vi "坐标映射.vi"(10 "位置":enum16{"A", "B", "C", "D", "E", "F", "G", "H"}(ring)) -> (0 "差值坐标":cluster{"X":i32, "Y":i32}, 1 "O均值坐标":cluster{"X":i32, "Y":i32}, 2 "位置均值坐标":cluster{"X":i32, "Y":i32}, 3 "位置坐标":cluster{"X":i32, "Y":i32}[](array[cluster]))   [LabVIEW 2015]
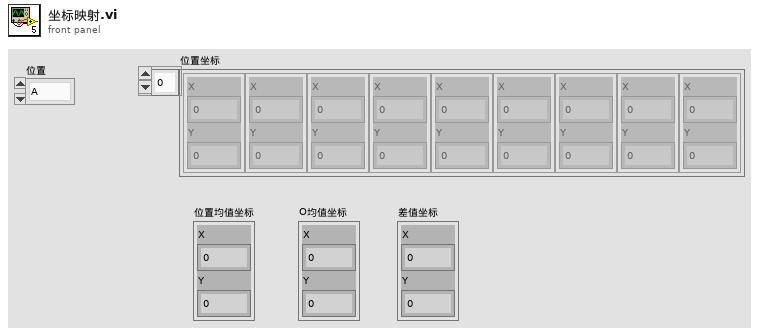
[diagram p1: front panel]
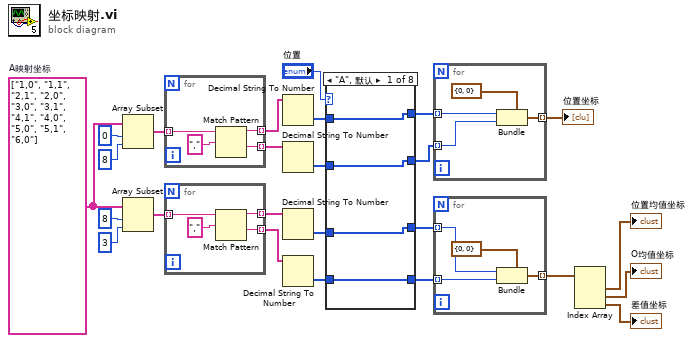
[diagram p0: block diagram]
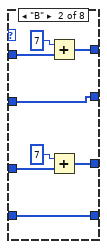
[diagram p2: hidden frame]
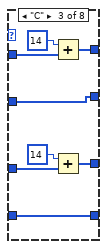
[diagram p3: hidden frame]
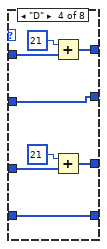
[diagram p4: hidden frame]
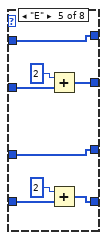
[diagram p5: hidden frame]
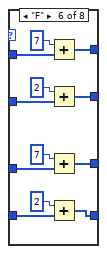
[diagram p6: hidden frame]
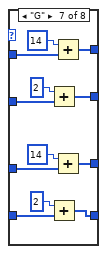
[diagram p7: hidden frame]
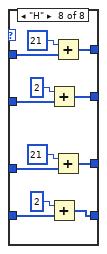
[diagram p8: hidden frame]
diagram:
  w16 = string[] ["1,0", "1,1", "2,1", "2,0", "3,0", "3,1", "4,1", "4,0", "5,0", "5,1", "6,0"]  # A映射坐标
  n1 = Array Subset(array=w16, index=0 ("索引"), length=8 ("索引")) -> (w15:string[])
  n2 = Array Subset(array=w16, index=8 ("索引"), length=3 ("索引")) -> (w14:string[])
  n3 = for {
    tunnel: w15 -> [w29] mode=indexing
    tunnel: [w27] -> w25 mode=indexing
    tunnel: [w26] -> w24 mode=indexing
    n4 = Match Pattern(string=w29, regular expression="," ("正则表达式")) -> (before substring=w27:string, after substring=w26:string)  [unwired: 1 in, 2 out]
  }
  n5 = for {
    tunnel: w14 -> [w33] mode=indexing
    tunnel: [w31] -> w13 mode=indexing
    tunnel: [w30] -> w12 mode=indexing
    n6 = Match Pattern(string=w33, regular expression="," ("正则表达式")) -> (before substring=w31:string, after substring=w30:string)  [unwired: 1 in, 2 out]
  }
  n7 = Decimal String To Number(string=w25) -> (number=w22:i32[])  [unwired: 2 in, 1 out]
  n8 = Decimal String To Number(string=w24) -> (number=w21:i32[])  [unwired: 2 in, 1 out]
  n9 = Decimal String To Number(string=w13) -> (number=w11:i32[])  [unwired: 2 in, 1 out]
  n10 = Decimal String To Number(string=w12) -> (number=w10:i32[])  [unwired: 2 in, 1 out]
  n11 = case shown="\"A\", 默认" "位置" {
    tunnel: [w37 w42 w50 w58 w69 w79 w91 w103] -> w3
    tunnel: w22 -> [w37 w44 w52 w60 w69 w81 w93 w105]
    tunnel: w21 -> [w36 w45 w53 w61 w67 w77 w89 w101]
    tunnel: [w36 w45 w53 w61 w66 w76 w88 w100] -> w2
    tunnel: w11 -> [w35 w40 w48 w56 w62 w73 w85 w97]
    tunnel: w10 -> [w34 w38 w46 w54 w64 w71 w84 w95]
    tunnel: [w35 w39 w47 w55 w62 w72 w83 w96] -> w9
    tunnel: [w34 w38 w46 w54 w63 w70 w82 w94] -> w8
    frame "A", Default {
    }
    frame "B" {
      n12 = Add(x=7, y=w44) -> (x+y=w42:i32[])
      n13 = Add(x=7, y=w40) -> (x+y=w39:i32[])
    }
    frame "C" {
      n14 = Add(x=14, y=w52) -> (x+y=w50:i32[])
      n15 = Add(x=14, y=w48) -> (x+y=w47:i32[])
    }
    frame "D" {
      n16 = Add(x=21, y=w60) -> (x+y=w58:i32[])
      n17 = Add(x=21, y=w56) -> (x+y=w55:i32[])
    }
    frame "E" {
      n18 = Add(x=2, y=w67) -> (x+y=w66:i32[])
      n19 = Add(x=2, y=w64) -> (x+y=w63:i32[])
    }
    frame "F" {
      n20 = Add(x=7, y=w81) -> (x+y=w79:i32[])
      n21 = Add(x=2, y=w77) -> (x+y=w76:i32[])
      n22 = Add(x=7, y=w73) -> (x+y=w72:i32[])
      n23 = Add(x=2, y=w71) -> (x+y=w70:i32[])
    }
    frame "G" {
      n24 = Add(x=2, y=w89) -> (x+y=w88:i32[])
      n25 = Add(x=2, y=w84) -> (x+y=w82:i32[])
      n26 = Add(x=14, y=w93) -> (x+y=w91:i32[])
      n27 = Add(x=14, y=w85) -> (x+y=w83:i32[])
    }
    frame "H" {
      n28 = Add(x=2, y=w101) -> (x+y=w100:i32[])
      n29 = Add(x=2, y=w95) -> (x+y=w94:i32[])
      n30 = Add(x=21, y=w105) -> (x+y=w103:i32[])
      n31 = Add(x=21, y=w97) -> (x+y=w96:i32[])
    }
  }
  n32 = for {
    tunnel: w3 -> [w109] mode=indexing
    tunnel: w2 -> [w108] mode=indexing
    tunnel: [w107] -> w1 mode=indexing
    n33 = Bundle(cluster=cluster{"X":i32, "Y":i32} {"X"=0, "Y"=0}, "X"=w109, "Y"=w108) -> (w107:cluster{"X":i32, "Y":i32})
  }
  "位置坐标" <- w1
  n34 = for {
    tunnel: w9 -> [w113] mode=indexing
    tunnel: w8 -> [w112] mode=indexing
    tunnel: [w111] -> w7 mode=indexing
    n35 = Bundle(cluster=cluster{"X":i32, "Y":i32} {"X"=0, "Y"=0}, "X"=w113, "Y"=w112) -> (w111:cluster{"X":i32, "Y":i32})
  }
  n36 = Index Array(array=w7) -> (element #1=→"位置均值坐标":cluster{"X":i32, "Y":i32}, element #2=→"O均值坐标":cluster{"X":i32, "Y":i32}, element #3=→"差值坐标":cluster{"X":i32, "Y":i32})  [unwired: 3 in]
